vi "Switching Levels Logic.vi"(6 "Hatch":bool, 7 "Cargo":bool, 8 "error in (no error)":errorcluster, 9 "Down":bool, 10 "Up":bool, 11 "Elevator in":refnum<class "Elevator.lvclass">) -> (0 "error out":errorcluster, 2 "Cargo/Hatch":T1, 3 "Elevator out":refnum<class "Elevator.lvclass">)   [LabVIEW 2018, in "Elevator.lvlib" / "Elevator.lvclass"]
uses:
  Elevator.lvclass
  Controls/Elevator Position.ctl
  Elevator.lvclass/Elevator.ctl
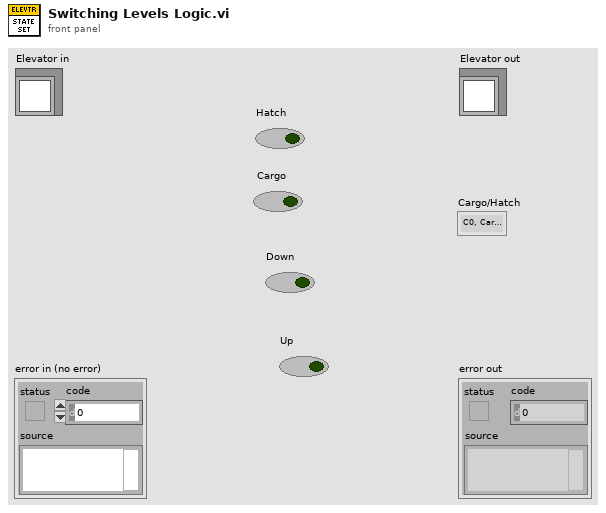
[diagram p1: front panel]
types:
  T1 = typedef "Elevator.lvlib/Elevator.lvclass/Elevator Position.ctl" = enum16{"C0, Cargo Ground", "C1, LV1 Cargo", "C2, Cargo Ship Cargo", "H0, LV1 Hatch", "H1, LV2 Hatch"}
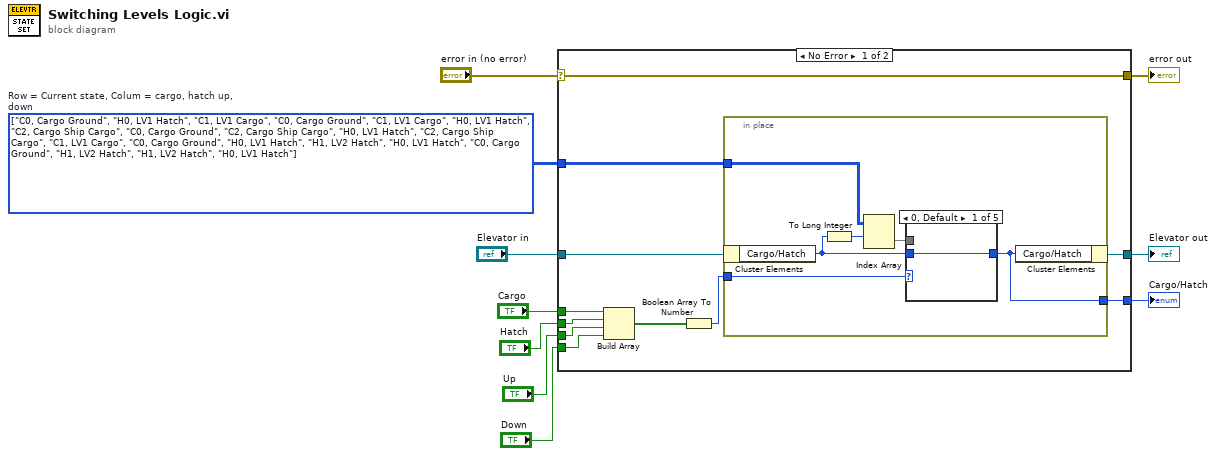
[diagram p0: block diagram]
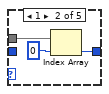
[diagram p2: hidden frame]
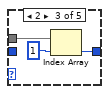
[diagram p3: hidden frame]
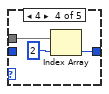
[diagram p4: hidden frame]
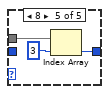
[diagram p5: hidden frame]
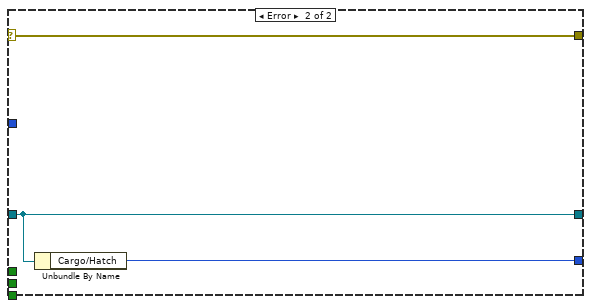
[diagram p6: hidden frame]
diagram:
  w6 = T1[][] [[enum."C0, Cargo Ground", enum."H0, LV1 Hatch", enum."C1, LV1 Cargo", enum."C0, Cargo Ground"], [enum."C1, LV1 Cargo", enum."H0, LV1 Hatch", enum."C2, Cargo Ship Cargo", enum."C0, Cargo Ground"], [enum."C2, Cargo Ship Cargo", enum."H0, LV1 Hatch", enum."C2, Cargo Ship Cargo", enum."C1, LV1 Cargo"], [enum."C0, Cargo Ground", enum."H0, LV1 Hatch", enum."H1, LV2 Hatch", enum."H0, LV1 Hatch"], [enum."C0, Cargo Ground", enum."H1, LV2 Hatch", enum."H1, LV2 Hatch", enum."H0, LV1 Hatch"]] items=["C0, Cargo Ground", "C1, LV1 Cargo", "C2, Cargo Ship Cargo", "H0, LV1 Hatch", "H1, LV2 Hatch"]  # Row = Current state, Colum = cargo, hatch up, down
  n1 = case shown="No Error" "error in (no error)" {
    selector: "error in (no error)" -> [w21 w43]
    tunnel: [w21 w43] -> w9
    tunnel: [w19 w42] -> w7
    tunnel: "Elevator in" -> [w20 w42]
    tunnel: w6 -> [w18 _]
    tunnel: "Up" -> [w12 _]
    tunnel: "Down" -> [w13 _]
    tunnel: "Cargo" -> [w14 _]
    tunnel: [w15 w41] -> w2
    tunnel: "Hatch" -> [w11 _]
    frame No Error {
      n2 = Build Array(w14, w11, w12, w13) -> (w17:bool[])
      n3 = Boolean Array To Number(Boolean array=w17) -> (number=w16:u32)
      n4 = in-place {
        in-place-border: w18 -> [w27]
        in-place-border: w16 -> [w25]
        in-place-border: [w22] -> w15
        n5 = in-place-cluster #1(w20) -> ("Cargo/Hatch"=w26:T1)
        n6 = To Long Integer(number=w26) -> (32bit integer=w24:i32)
        n7 = Index Array(array=w27, index (row)=w24) -> (element=w23:T1[])  [unwired: 1 in]
        n8 = case shown="0, Default" w25 {
          tunnel: w26 -> [w28 _ _ _ _]
          tunnel: [w28 w31 w34 w37 w40] -> w22
          tunnel: w23 -> [_ w30 w33 w36 w39]
          frame 0, Default {
          }
          frame 1 {
            n9 = Index Array(array=w30, index=0) -> (element=w31:T1)
          }
          frame 2 {
            n10 = Index Array(array=w33, index=1) -> (element=w34:T1)
          }
          frame 4 {
            n11 = Index Array(array=w36, index=2) -> (element=w37:T1)
          }
          frame 8 {
            n12 = Index Array(array=w39, index=3) -> (element=w40:T1)
          }
        }
        n13 = in-place-cluster #1("Cargo/Hatch"=w22) -> (w19:refnum<class "Elevator.lvclass">)
      }
    }
    frame Error {
      n14 = Unbundle By Name(w42) -> ("Cargo/Hatch"=w41:T1)
    }
  }
  "error out" <- w9
  "Elevator out" <- w7
  "Cargo/Hatch" <- w2
